vi "niRFUtil ERR Check Valid RBW Definition.vi"(0 "Filter Type":T2=enum."Gaussian", 7 "Bandwidth Definition":T1, 11 "error in (no error)":errorcluster) -> (15 "error out":errorcluster)   [LabVIEW 2015, in "niRFUtil.lvlib"]
uses:
  niRFUtil.lvlib
  Includes/niRFUtil INC RBW Filter Type (Freq Domain).ctl
  Includes/niRFUtil INC Bandwidth Definition.ctl
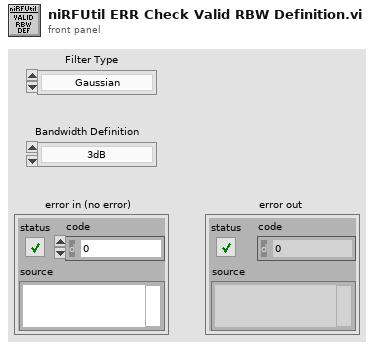
[diagram p1: front panel]
types:
  T1 = typedef "niRFUtil.lvlib/niRFUtil INC Bandwidth Definition.ctl" = enum16{"3dB", "6dB", "Bin Width", "ENBW"}
  T2 = typedef "niRFUtil.lvlib/niRFUtil INC RBW Filter Type (Freq Domain).ctl" = enum16{"FFT Based", "Gaussian", "Flat", "Synch Tuned - 4", "Synch Tuned - 5"}
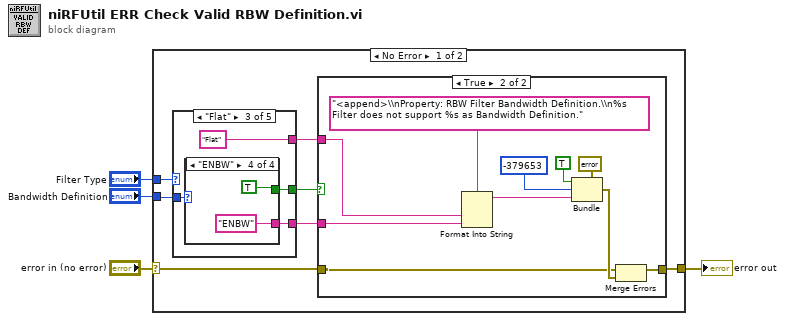
[diagram p0: block diagram]
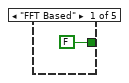
[diagram p3: hidden frame]
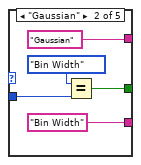
[diagram p4: hidden frame]
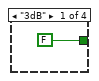
[diagram p5: hidden frame]
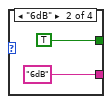
[diagram p6: hidden frame]
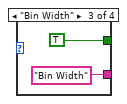
[diagram p7: hidden frame]
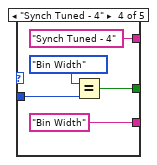
[diagram p8: hidden frame]
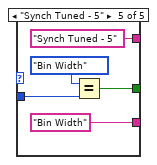
[diagram p9: hidden frame]
diagram:
  n1 = case shown="No Error" "error in (no error)" {
    selector: "error in (no error)" -> [w7 w50]
    tunnel: [w11 w50] -> w4
    tunnel: "Bandwidth Definition" -> [w8 _]
    tunnel: "Filter Type" -> [w9 _]
    frame No Error {
      n2 = case shown="\"Flat\"" w9 {
        tunnel: w8 -> [_ w28 w32 w44 w49]
        tunnel: [FALSE w26 w31 w42 w47] -> w10
        tunnel: [_ "Bin Width" ("element") w30 "Bin Width" ("element") "Bin Width" ("element")] -> w6
        tunnel: [_ "Gaussian" ("element") "Flat" ("element") "Synch Tuned - 4" ("element") "Synch Tuned - 5" ("element")] -> w5
        frame "FFT Based" {
        }
        frame "Gaussian" {
          n3 = Equal?(x=niRFUtil_INC_Bandwidth_Definition."Bin Width", y=w28) -> (x = y?=w26:bool)
        }
        frame "Flat" {
          n4 = case shown="\"ENBW\"" w32 {
            tunnel: [FALSE TRUE TRUE TRUE] -> w31
            tunnel: [_ "6dB" ("element") "Bin Width" ("element") "ENBW" ("element")] -> w30
            frame "3dB" {
            }
            frame "6dB" {
            }
            frame "Bin Width" {
            }
            frame "ENBW" {
            }
          }
        }
        frame "Synch Tuned - 4" {
          n5 = Equal?(x=niRFUtil_INC_Bandwidth_Definition."Bin Width", y=w44) -> (x = y?=w42:bool)
        }
        frame "Synch Tuned - 5" {
          n6 = Equal?(x=niRFUtil_INC_Bandwidth_Definition."Bin Width", y=w49) -> (x = y?=w47:bool)
        }
      }
      n7 = case shown="True" w10 {
        tunnel: [w12 w15] -> w11
        tunnel: w7 -> [w12 w13]
        tunnel: w6 -> [_ w21]
        tunnel: w5 -> [_ w20]
        frame False {
        }
        frame True {
          n8 = Format Into String(format string="<append>\\nProperty: RBW Filter Bandwidth Definition.\\n%s Filter does not support %s as Bandwidth Definition." ("initial string"), w20, w21) -> (resulting string=w17:string)  [unwired: 2 in, 1 out]
          n9 = Bundle(cluster=cluster{"status":bool, i32, string} {"status"=FALSE, 0, ""}, "status"=TRUE, -379653, w17) -> (w14:cluster{"status":bool, i32, string})
          n10 = Merge Errors(w13, w14) -> (w15:errorcluster)
        }
      }
    }
    frame Error {
    }
  }
  "error out" <- w4
